vi "Init2.vi"(8 "error in (no error)":errorcluster, 10 "Addresses":T1, 11 "TranslationStageActor in":refnum<class "ArduinoTranslationStage.lvclass">) -> (0 "error out":errorcluster, 3 "TranslationStageActor out":refnum<class "ArduinoTranslationStage.lvclass">)   [LabVIEW 2023, in "ArduinoTranslationStage.lvlib" / "ArduinoTranslationStage.lvclass"]
uses:
  ArduinoTranslationStage.lvclass
  ArduinoTranslationStage.lvclass/ArduinoTranslationStage.ctl
  Cameras_LV/InitDeinitComm Messages/InitDone Msg/InitDone Msg.lvclass
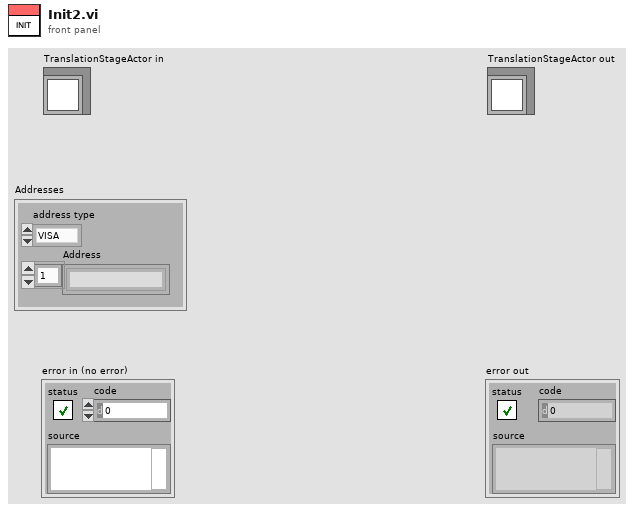
[diagram p1: front panel]
types:
  T1 = cluster{"address type":enum16{"VISA", "Index"}, "Address":string[]}
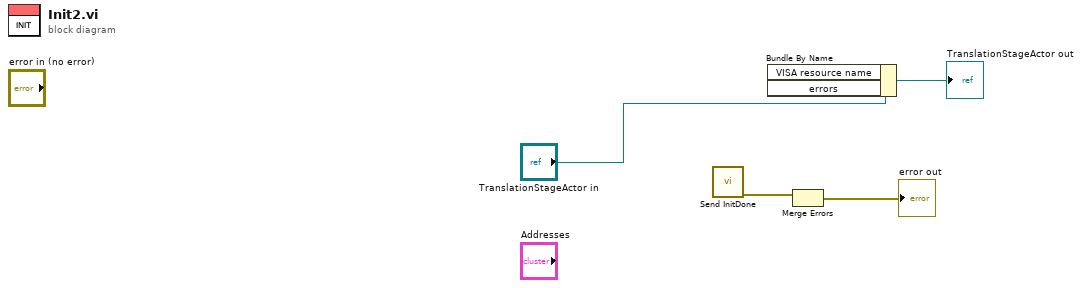
[diagram p0: block diagram]
diagram:
  n1 = call "Send InitDone.vi"() -> ("error out"=w1:errorcluster, "Message Enqueuer"=w2:refnum<class "Message Enqueuer.lvclass">)  [unwired: 9 in, 1 out]
  n2 = Bundle By Name(cluster="TranslationStageActor in") -> (→"TranslationStageActor out":refnum<class "ArduinoTranslationStage.lvclass">)  [unwired: 2 in]
  n3 = Merge Errors(w1) -> (→"error out":errorcluster)  [unwired: 1 in]
